vi "Stream Control.vi"() -> ()   [LabVIEW 2017]
panel:
  in  "Save":bool
  in  "Decimations":cluster{"Decimation":u32}[](array[cluster])=[{"Decimation"=200}, {"Decimation"=40}, {"Decimation"=40}, {"Decimation"=2}, {"Decimation"=2}]
  out "Master frequency":dbl[unit]=800.0
  out "Stream":cluster{"Name":string, "Rate":dbl[unit]}[](array[cluster])=[{"Name"="gmr", "Rate"=200.0}, {"Name"="accel", "Rate"=40.0}, {"Name"="gyro", "Rate"=40.0}, {"Name"="bar", "Rate"=2.0}, {"Name"="therm", "Rate"=2.0}]
  in  "URL":refnum<visa-resource-name>="ASRL15::INSTR"
  in  "Quit":bool
  out "ID":string="Twinleaf VMR R9 [DEV]"
  # "Stream Control"
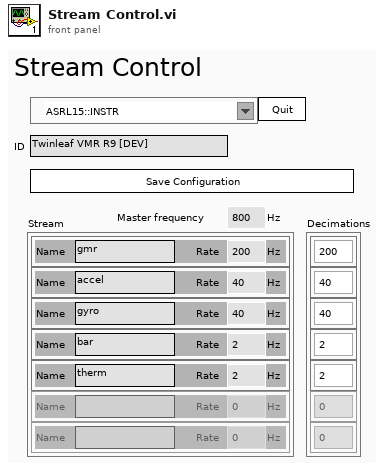
[diagram p1: front panel]
types:
  T1 = cluster{"TS Connection":cluster{"Type":enum16{"Serial", "TCP", "UDP", "mUDP"}, "URL":refnum<visa-resource-name>, "TO":u32, "Addr":u32, "Port":i32, "TCP":refnum<k5>, "UDP":refnum<k16>, "Route":string}, "REQ":refnum<queue>, "REP":refnum<queue>}
  T2 = cluster{"Awaiting REP":bool, "REQ ID":u32, "dstreams in":cluster{"id":u16, "timebase id":u16, "period":u32, "offset":u32, "sample number":u64, "total components":u16, "flags":u16, "components":cluster{"pstream id":u16, "flags":u16, "period":u32, "offset":u32}[]}[], "pstreams":cluster{"id":u16, "timebase_id":u16, "period":u32, "offset":u32, "fmt":i32, "flags":u16, "channels":u16, "type":u8, "name":string, "column names":string[], "title":string, "units":string}[], "timebases":cluster{"id":u16, "source":u8, "epoch":u8, "start time":u64, "period numerator (µs)":u32, "period denominator (µs)":u32, "flags":u32, "stability":sgl, "source id":string}[]}
  T3 = cluster{"TC Connection":cluster{"Type":enum16{"Serial", "TCP", "UDP", "mUDP"}, "URL":refnum<visa-resource-name>, "TO":u32, "Addr":u32, "Port":i32, "TCP":refnum<k5>, "UDP":refnum<k16>, "Route":string}, "REQ":refnum<queue>, "REP":refnum<queue>}
  T4 = cluster{"id":u16, "source":u8, "epoch":u8, "start time":u64, "period numerator (µs)":u32, "period denominator (µs)":u32, "flags":u32, "stability":sgl, "source id":string}[]
  T5 = cluster{"id":u16, "timebase_id":u16, "period":u32, "offset":u32, "fmt":i32, "flags":u16, "channels":u16, "type":u8, "name":string, "column names":string[], "title":string, "units":string}[]
  T6 = cluster{"id":u16, "timebase id":u16, "period":u32, "offset":u32, "sample number":u64, "total components":u16, "flags":u16, "components":cluster{"pstream id":u16, "flags":u16, "period":u32, "offset":u32}[]}[]
  T7 = cluster{"id":u16, "timebase id":u16, "period":u32, "offset":u32, "sample number":u64, "total components":u16, "flags":u16, "components":cluster{"pstream id":u16, "flags":u16, "period":u32, "offset":u32}[]}
  T8 = cluster{"pstream id":u16, "flags":u16, "period":u32, "offset":u32}[]
  T9 = cluster{"id":u16, "source":u8, "epoch":u8, "start time":u64, "period numerator (µs)":u32, "period denominator (µs)":u32, "flags":u32, "stability":sgl, "source id":string}
  T10 = cluster{"id":u16, "timebase_id":u16, "period":u32, "offset":u32, "fmt":i32, "flags":u16, "channels":u16, "type":u8, "name":string, "column names":string[], "title":string, "units":string}
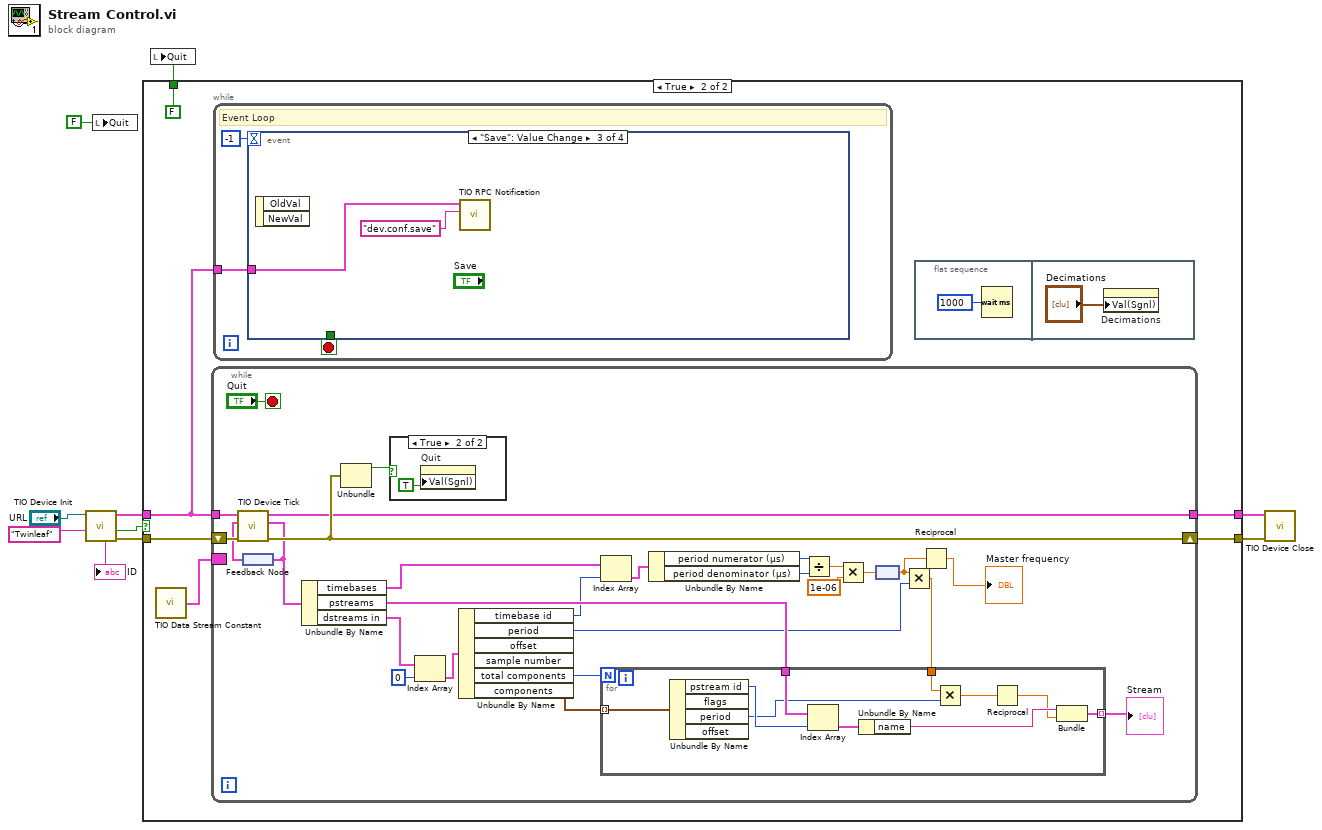
[diagram p0: block diagram]
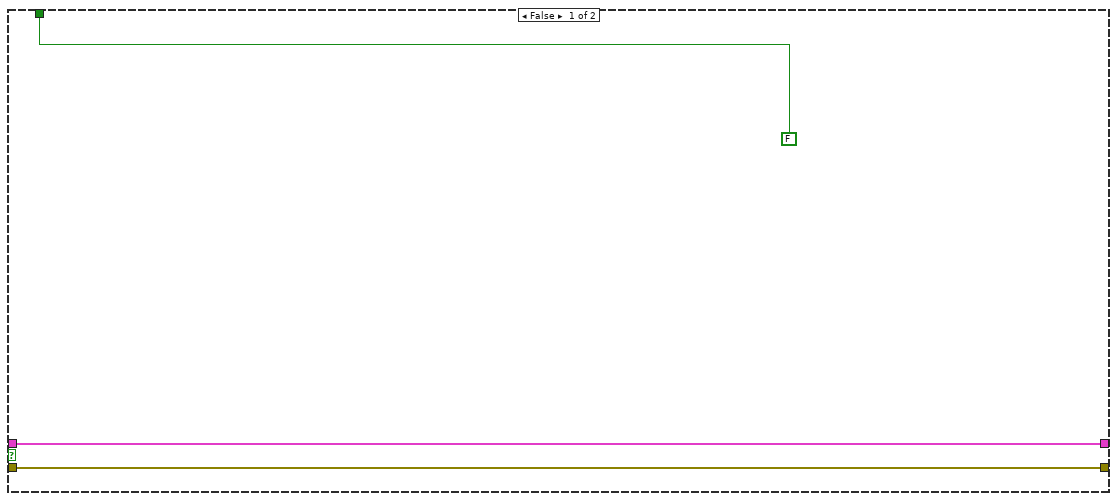
[diagram p2: hidden frame]
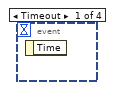
[diagram p4: hidden frame]
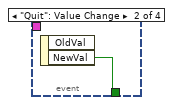
[diagram p5: hidden frame]
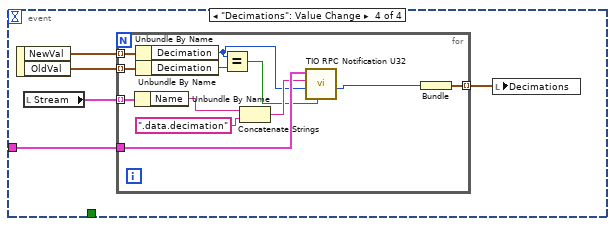
[diagram p6: hidden frame]
diagram:
  n1 = call "TIO Device Init.vi"("ID"="Twinleaf" ("Prefix"), "URL"="URL") -> ("error out"=w9:errorcluster, "Connected"=w1:bool, "TIO"=w10:T1, "ID Verified"=→"ID":string)  [unwired: 5 in, 1 out]
  n2 = local write "Quit"(FALSE ("Kill")) -> ()
  n3 = case shown="True" w1 {
    tunnel: w10 -> [w12 w18]
    tunnel: w9 -> [w11 w19]
    tunnel: [FALSE FALSE ("Kill")] -> w5
    tunnel: [w12 w16] -> w3
    tunnel: [w11 w15] -> w4
    frame False {
    }
    frame True {
      n4 = call "TIO Data Stream Constant.vi"() -> ("TIO State"=w14:T2)
      n5 = while {
        tunnel: w18 -> [w48]
        border: w14 -> [_]
        tunnel: [w42] -> w16
        shift-right: [w44] -> w15
        shift-left: w19 -> [w47]
        stop <- "Quit" stop-if-true
        n6 = feedback #1() -> (w45:T2)
        n7 = call "TIO Device Tick.vi"("Error in"=w47, "TIO State"=w45, "TIO"=w48) -> ("Error out"=w44:errorcluster, "TIO State"=w27:T2, "TIO"=w42:T3)  [unwired: 5 in, 1 out]
        n8 = feedback-in #1(w27) -> ()
        n9 = Unbundle By Name(w27) -> ("timebases"=w34:T4, "pstreams"=w36:T5, "dstreams in"=w40:T6)
        n10 = Unbundle(w44) -> ("status"=w43:bool)  [unwired: 2 out]
        n11 = case shown="True" w43 {
          frame False {
          }
          frame True {
            n12 = property on="Quit" class="Bool (strict)"("Val(Sgnl)"=TRUE ("Value (Signaling)")) -> ()  [unwired: 2 in, 2 out]
          }
        }
        n13 = Index Array(array=w40, index=0) -> (element=w39:T7)
        n14 = Unbundle By Name(w39) -> ("timebase id"=w35:u16, "period"=w23:u32, "total components"=w38:u16, "components"=w37:T8)  [unwired: 2 out]
        n15 = Index Array(array=w34, index=w35) -> (element=w33:T9)
        n16 = Unbundle By Name(w33) -> ("period numerator (µs)"=w32:u32, "period denominator (µs)"=w31:u32)
        n17 = Divide(x=w32, y=w31) -> (x/y=w30:dbl)
        n18 = Multiply(x=w30, y=1e-06) -> (x*y=w26:dbl)
        n19 = node(w26) -> (w25:dbl[unit])
        n20 = Multiply(x=w25, y=w23) -> (x*y=w28:dbl[unit])
        n21 = for {
          N: w38 -> [_]
          tunnel: w37 -> [w58] mode=indexing
          tunnel: w36 -> [w56]
          tunnel: w28 -> [w57]
          tunnel: [w52] -> w22 mode=indexing
          n22 = Unbundle By Name(w58) -> ("pstream id"=w55:u16, "period"=w50:u32)  [unwired: 2 out]
          n23 = Index Array(array=w56, index=w55) -> (element=w54:T10)
          n24 = Unbundle By Name(w54) -> ("name"=w53:string)
          n25 = Multiply(x=w57, y=w50) -> (x*y=w49:dbl[unit])
          n26 = Reciprocal(x=w49) -> (1/x=w51:dbl[unit])
          n27 = Bundle("name"=w53, w51) -> (w52:cluster{"name":string, dbl[unit]})  [unwired: 1 in]
        }
        "Stream" <- w22
        n28 = Reciprocal(x=w25) -> (1/x=→"Master frequency":dbl[unit])
      }
      n29 = while {
        tunnel: w18 -> [w61]
        stop <- w60 stop-if-true
        # "Event Loop"
        n30 = event shown="[2] \"Save\": Value Change" {
          selector: _ -> [_ _ _ _]
          dyn-events: _ -> [_ _ _ _]
          timeout: -1 -> [_ _ _ _]
          tunnel: w61 -> [_ _ w64 w67]
          tunnel: [_ w63 _ _] -> w60
          event Timeout {
            n31 = event-data() -> ()  [unwired: 1 in, 1 out]
          }
          event "Quit": Value Change {
            n32 = event-data() -> ("NewVal"=w63:bool)  [unwired: 1 in, 1 out]
          }
          event "Save": Value Change {
            n33 = event-data() -> ()  [unwired: 1 in, 2 out]
            n34 = call "TIO RPC Notification.vi"("Topic"="dev.conf.save" ("String"), "TIO"=w64) -> ()  [unwired: 6 in, 3 out]
          }
          event "Decimations": Value Change {
            n35 = event-data() -> ("NewVal"=w70:cluster{"Decimation":u32}[], "OldVal"=w69:cluster{"Decimation":u32}[])  [unwired: 1 in]
            n36 = local read "Stream"() -> (w68:cluster{"Name":string, "Rate":dbl[unit]}[])
            n37 = for {
              tunnel: w70 -> [w82] mode=indexing
              tunnel: w69 -> [w81] mode=indexing
              tunnel: w68 -> [w79] mode=indexing
              tunnel: w67 -> [w76]
              tunnel: [w71] -> w66 mode=indexing
              n38 = Unbundle By Name(w79) -> ("Name"=w78:string)
              n39 = Unbundle By Name(w82) -> ("Decimation"=w73:u32)
              n40 = Unbundle By Name(w81) -> ("Decimation"=w80:u32)
              n41 = Equal?(x=w73, y=w80) -> (x = y?=w74:bool)
              n42 = Concatenate Strings(w78, ".data.decimation") -> (w75:string)
              n43 = call "TIO RPC Notification U32.vi"("Read"=w74, "Set value"=w73, "Topic"=w75, "TIO"=w76) -> ("Get value (default if error)"=w72:u32)  [unwired: 4 in, 2 out]
              n44 = Bundle("Get value (default if error)"=w72) -> (w71:cluster{"Get value (default if error)":u32})  [unwired: 1 in]
            }
            n45 = local write "Decimations"(w66) -> ()
          }
        }
      }
      n46 = flat-sequence {
        frame #0 {
          n47 = Wait (ms)(milliseconds to wait=u32 1000) -> ()  [unwired: 1 out]
        }
        frame #1 {
          n48 = property on="Decimations" class="Arr (strict)"("Val(Sgnl)"="Decimations") -> ()  [unwired: 2 in, 2 out]
        }
      }
    }
  }
  n49 = local write "Quit"(w5) -> ()
  n50 = call "TIO Device Close.vi"("Error in"=w4, "TIO"=w3) -> ()  [unwired: 10 in]
